vi "While Loop Basics.vi"() -> ()   [LabVIEW 2020]
panel:
  out "Hours":dbl
  out "Minutes":dbl
  out "Seconds":dbl
  out "Iteration":i32
  in  "Stop":bool
  in  "Total Time in Seconds":dbl
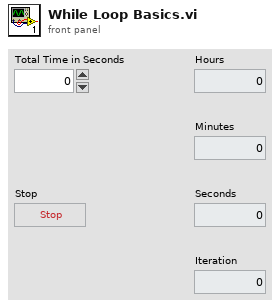
[diagram p1: front panel]
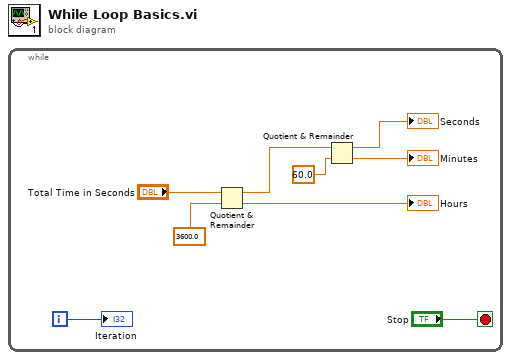
[diagram p0: block diagram]
diagram:
  n1 = while {
    i -> [w2]
    stop <- "Stop" stop-if-true
    n2 = Quotient & Remainder(x="Total Time in Seconds", y=3600.0) -> (x-y*floor(x/y)=w7:dbl, floor(x/y)=→"Hours":dbl)
    n3 = Quotient & Remainder(x=w7, y=60.0) -> (x-y*floor(x/y)=→"Seconds":dbl, floor(x/y)=→"Minutes":dbl)
    "Iteration" <- w2
  }
